vi "Load_Boston.vi"(8 "error in":errorcluster caption="entrée d'erreur") -> (0 "error out":errorcluster caption="sortie d'erreur", 3 "Tableau":string[][](array[string]))   [LabVIEW 2020]
doc: "Data Set Characteristics :\n\nNumber of Instances : 506\n\nNumber of Attributes : 13 numeric/categorical predictive. Median Value (attribute 14) is usually the target.\n\nAttribute Information (in order)\n\n- CRIM per capita crime rate by town\n- ZN proportion of residential land zoned for lots over 25,000 sq.ft.\n- INDUS proportion of non-retail business acres per town\n- CHAS Charles River dummy variable (= 1 if tract bounds river; 0 otherwise)\n- NOX nitric oxides concentration (parts per 10 million)\n- RM average number of rooms per dwelling\n- AGE proportion of owner-occupied units built prior to 1940\n- DIS weighted distances to five Boston employment centres\n- RAD index of accessibility to radial highways\n- TAX full-value property-tax rate per $10,000\n- PTRATIO pupil-teacher ratio by town\n- B 1000(Bk - 0.63)^2 where Bk is the proportion of blacks by town\n- LSTAT % lower status of the population\n- MEDV Median value of owner-occupied homes in $1000’s\n\nMissing Attribute Values : None\n\nCreator : Harrison, D. and Rubinfeld, D.L.\n\n\n\n\nThis dataset was taken from the StatLib library which is maintained at Carnegie Mellon University.\n\nThe Boston house-price data of Harrison, D. and Rubinfeld, D.L. ‘Hedonic prices and the demand for clean air’, J. Environ. Economics & Management, vol.5, 81-102, 1978. Used in Belsley, Kuh & Welsch, ‘Regression diagnostics …’, Wiley, 1980. N.B. Various transformations are used in the table on pages 244-261 of the latter.\n\nThe Boston house-price data has been used in many machine learning papers that address regression problems."
uses:
  Load_Boston.lvclass
panel:
  out "Load_Boston en sortie":refnum<class "Load_Boston.lvclass">
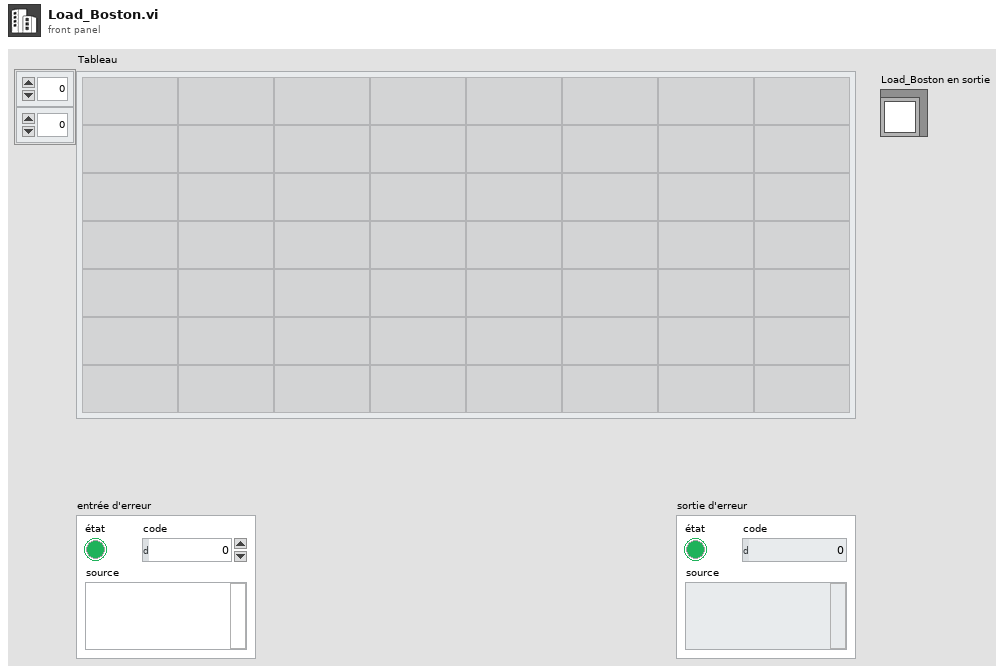
[diagram p1: front panel]
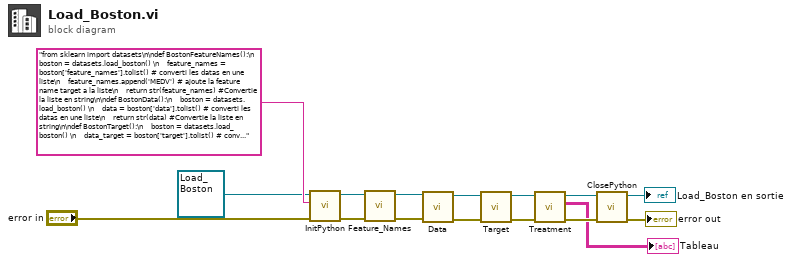
[diagram p0: block diagram]
diagram:
  n1 = call-dynamic "InitPython.vi"("error in (no error)"="error in", "Python Instruction"="from sklearn import datasets\n\ndef BostonFeatureNames():\n    boston = datasets.load_boston() \n    feature_names = boston['feature_names'].tolist() # converti les datas en une liste\n    feature_names.append('MEDV') # ajoute la feature name target a la liste\n    return str(feature_names) #Convertie la liste en string\n\ndef BostonData():\n    boston = datasets.load_boston() \n    data = boston['data'].tolist() # converti les datas en une liste\n    return str(data) #Convertie la liste en string\n\ndef BostonTarget():\n    boston = datasets.load_boston() \n    data_target = boston['target'].tolist() # converti les datas en une liste\n    return str(data_target) #Convertie la liste en string", "Scikit-learn en entrée"=refnum<class "Load_Boston.lvclass"> refnum ("Load_Boston.lvclass")) -> ("error out"=w13:errorcluster, "Scikit-learn en sortie"=w6:refnum<class "Load_Boston.lvclass">)  [unwired: 7 in]
  n2 = call-dynamic "Feature_Names.vi"("error in (no error)"=w13, "Load_Boston en entrée"=w6) -> ("error out"=w11:errorcluster, "Load_Boston en sortie"=w12:refnum<class "Load_Boston.lvclass">)  [unwired: 8 in]
  n3 = call-dynamic "Data.vi"("error in (no error)"=w11, "Load_Boston en entrée"=w12) -> ("error out"=w4:errorcluster, "Load_Boston en sortie"=w5:refnum<class "Load_Boston.lvclass">)  [unwired: 8 in]
  n4 = call-dynamic "Target.vi"("error in (no error)"=w4, "Load_Boston en entrée"=w5) -> ("error out"=w2:errorcluster, "Load_Boston en sortie"=w3:refnum<class "Load_Boston.lvclass">)  [unwired: 8 in]
  n5 = call-dynamic "Treatment.vi"("error in (no error)"=w2, "Load_Boston en entrée"=w3) -> ("error out"=w10:errorcluster, "Tableau"=→"Tableau":string[][], "Load_Boston en sortie"=w9:refnum<class "Load_Boston.lvclass">)  [unwired: 7 in]
  n6 = call-dynamic "ClosePython.vi"("error in (no error)"=w10, "Scikit-learn en entrée"=w9) -> ("error out"=→"error out":errorcluster, "Scikit-learn en sortie"=→"Load_Boston en sortie":refnum<class "Load_Boston.lvclass">)  [unwired: 8 in]
